vi "dist btwn 2 points.vi"(10 "coord pair 2":dbl[](array[numeric]), 11 "coord pair1":dbl[](array[numeric])) -> (3 "dist":dbl)   [LabVIEW 2019]
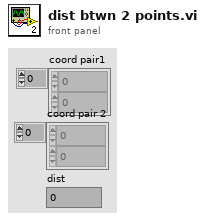
[diagram p1: front panel]
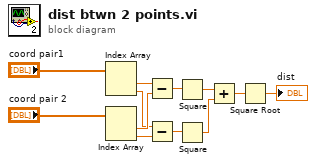
[diagram p0: block diagram]
diagram:
  n1 = Index Array(array="coord pair1") -> (element #1=w4:dbl, element #2=w2:dbl)  [unwired: 2 in]
  n2 = Index Array(array="coord pair 2") -> (element #1=w3:dbl, element #2=w1:dbl)  [unwired: 2 in]
  n3 = Subtract(x=w4, y=w3) -> (x-y=w12:dbl)
  n4 = Subtract(x=w2, y=w1) -> (x-y=w11:dbl)
  n5 = Square(x=w12) -> (x^2=w10:dbl)
  n6 = Square(x=w11) -> (x^2=w9:dbl)
  n7 = Add(x=w10, y=w9) -> (x+y=w8:dbl)
  n8 = Square Root(x=w8) -> (sqrt(x)=→"dist":dbl)
